vi "HP34401_config_4wR.vi"(7 "Manual Range (1.00)":dbl, 8 "error in":errorcluster, 11 "VISA in":refnum<visa-resource-name>) -> (0 "error out":errorcluster, 3 "VISA out":refnum<visa-resource-name>)   [LabVIEW 2020]
uses:
  drivers/HP34401A/Agilent 34401.lvlib
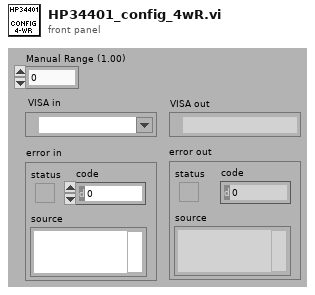
[diagram p1: front panel]
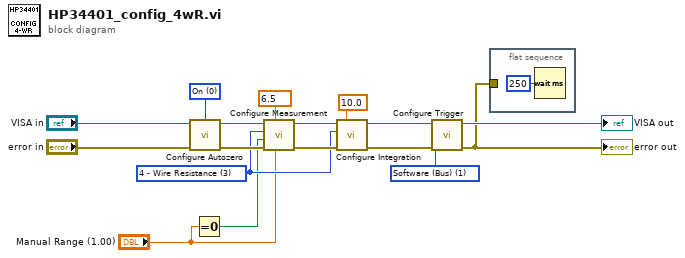
[diagram p0: block diagram]
diagram:
  w3 = 10.0 items=["0.001"=0.001, "0.002"=0.002, "0.006"=0.006, "0.02"=0.02, "0.06"=0.06, "0.2"=0.2, "1"=1.0, "10"=10.0, "100"=100.0] ("Integration Time (1 PLCs)")
  w11 = u16 1 items=["Immediate", "Software (Bus)", "External", "Internal"] ("Trigger Source (0: Immediate)")
  w12 = u16 0 items=["On", "Off", "Once"] ("Autozero  (0: On)")
  w4 = u16 3 items=["DC Voltage", "AC Voltage", "2 - Wire Resistance", "4 - Wire Resistance", "DC Current", "AC Current", "Frequency", "Period", "Continuity", "Diode Checking", "VDC:VDC Ratio", "Temperature", "Capacitance"] ("Function (0: DC Voltage)")
  w17 = 6.5 items=["4.5"=4.5, "5.5"=5.5, "6.5"=6.5] ("Manual Resolution (5.5 Digits)")
  n1 = call "Configure Autozero.vi"("error in (no error)"="error in", "Autozero  (0: On)"=w12, "VISA resource name"="VISA in") -> ("error out"=w15:errorcluster, "VISA resource name out"=w14:refnum<visa-resource-name>)  [unwired: 7 in]
  n2 = Equal To 0?(x="Manual Range (1.00)") -> (x = 0?=w1:bool)
  n3 = call "Configure Measurement.vi"("Manual Range (1.00)"="Manual Range (1.00)", "Manual Resolution (5.5 Digits)"=w17, "error in (no error)"=w15, "Enable Auto Range (T: Enable)"=w1, "Function (0: DC Voltage)"=w4, "VISA resource name"=w14) -> ("error out"=w8:errorcluster, "VISA resource name out"=w7:refnum<visa-resource-name>)  [unwired: 4 in]
  n4 = call "Configure Integration.vi"("error in (no error)"=w8, "Integration Time (1 PLCs)"=w3, "Function (0: DC Voltage)"=w4, "VISA resource name"=w7) -> ("error out"=w5:errorcluster, "VISA resource name out"=w6:refnum<visa-resource-name>)  [unwired: 6 in]
  n5 = call "Configure Trigger.vi"("error in (no error)"=w5, "Trigger Source (0: Immediate)"=w11, "VISA resource name"=w6) -> ("error out"=w9:errorcluster, "VISA resource name out"=→"VISA out":refnum<visa-resource-name>)  [unwired: 7 in]
  "error out" <- w9
  n6 = flat-sequence {
    tunnel: w9 -> [_]
    frame #0 {
      n7 = Wait (ms)(milliseconds to wait=u32 250) -> ()  [unwired: 1 out]
    }
  }
